vi "Configure Sensing Threshold.vi"(5 "Threshold Level (0)":dbl, 7 "Threshold Operation (0: Greater Than)":u16(ring) items=["Greater Than", "Less Than"], 8 "error in (no error)":errorcluster, 9 "Sensing Function (3: Volt)":u16(ring)=3 items=["Amp-Hour", "Current", "Power", "Voltage", "Watt-Hour"], 10 "Comparator Number (1)":u16=1, 11 "VISA resource name":refnum<visa-resource-name>) -> (0 "error out":errorcluster, 3 "VISA resource name out":refnum<visa-resource-name>)   [LabVIEW 2019, in "Agilent N7976A.lvlib"]
doc: "Configures the threshold necessary for sensors."
uses:
  <instrlib>/Agilent N7976A/Agilent N7976A.lvlib
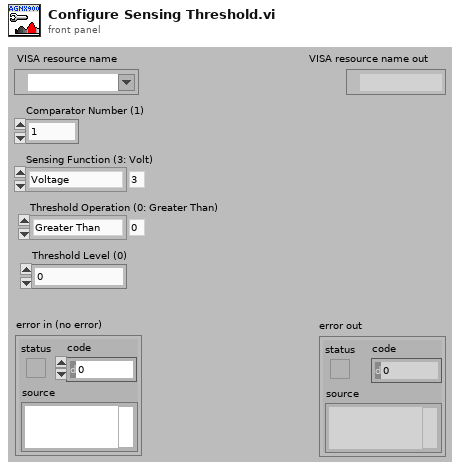
[diagram p1: front panel]
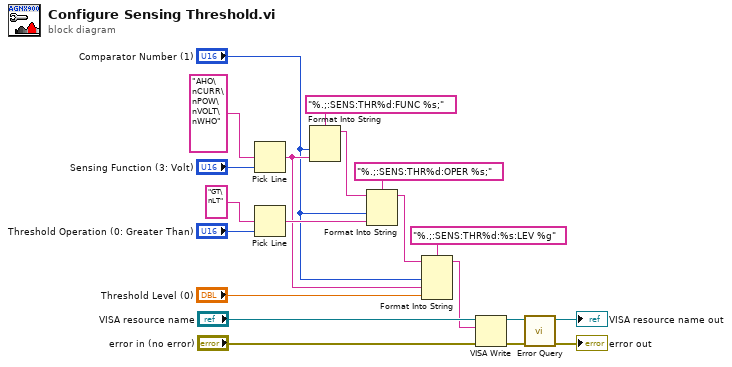
[diagram p0: block diagram]
diagram:
  n1 = Pick Line(multi-line string="AHO\nCURR\nPOW\nVOLT\nWHO", line index="Sensing Function (3: Volt)") -> (output string=w3:string)  [unwired: 1 in]
  n2 = Pick Line(multi-line string="GT\nLT", line index="Threshold Operation (0: Greater Than)") -> (output string=w5:string)  [unwired: 1 in]
  n3 = Format Into String(format string="%.;:SENS:THR%d:FUNC %s;", "Comparator Number (1)", w3) -> (resulting string=w4:string)  [unwired: 2 in, 1 out]
  n4 = Format Into String(format string="%.;:SENS:THR%d:OPER %s;", initial string=w4, "Comparator Number (1)", w5) -> (resulting string=w10:string)  [unwired: 1 in, 1 out]
  n5 = Format Into String(format string="%.;:SENS:THR%d:%s:LEV %g", initial string=w10, "Comparator Number (1)", w3, "Threshold Level (0)") -> (resulting string=w12:string)  [unwired: 1 in, 1 out]
  n6 = VISA Write(VISA resource name="VISA resource name", write buffer=w12, error in (no error)="error in (no error)") -> (VISA resource name out=w17:refnum<visa-resource-name>, error out=w18:errorcluster)  [unwired: 1 out]
  n7 = call <instrlib>:"Error Query.vi"("error in (no error)"=w18, "VISA resource name"=w17) -> ("error out"=→"error out":errorcluster, "VISA resource name out"=→"VISA resource name out":refnum<visa-resource-name>)  [unwired: 6 in, 2 out]
